vi "Set Center-Span.vi"() -> ()   [LabVIEW 2012, in "Microwave.lvclass"]
doc: "Sets the center and span (or start and stop) frequencies for a microwave sweep."
uses:
  Microwave.lvclass
  Microwave.lvclass/Microwave.ctl
  Math Operations/To Center and Span (frequency).vi
  Math Operations/To Start and Stop (frequency).vi
  Agilent PSG MXG Series/Agilent PSG MXG Series.lvlib
panel:
  in  "Adjust":bool
  in  "Distance from center\n(+/- # of boxes)":dbl
  in  "Width of scan\n(# of boxes)":dbl
  out "Ready when\nblinking":bool
  out "Dwell":dbl[unit]=0.052000000000000005 caption="Steps"
  in  "Dwell Set":dbl[unit]=0.001
  out "Steps":i32=52
  out "Power":dbl=23.0
  in  "Steps Set":i32=101
  in  "Power Set":dbl=23.0
  out "Current Amplitude Mode":enum16{"Fixed", "Stepped Sweep", "List Sweep"}(ring)
  out "Current Frequency Mode":T1(ring)
  out "error out":errorcluster
  in  "Copy actual to set":bool
  in  "Populate fields with member data":bool
  out "Fake Microwave out":refnum<class "Microwave.lvclass">
  in  "error in (no error)":errorcluster
  in  "Fake Microwave in":refnum<class "Microwave.lvclass">
  out "Stop":dbl[unit] caption="Center"
  in  "Stop Set":dbl[unit]
  out "Start":dbl[unit] caption="Center"
  in  "Start Set":dbl[unit]
  in  "Read to Control":bool
  in  "Read":bool
  out "Span":dbl[unit]
  out "Center":dbl[unit]
  in  "Span Set":dbl[unit] caption="Span"
  in  "Center Set":dbl[unit] caption="Center"
  in  "Rf On/Off":bool caption="RF On/Off"
  in  "Exit":bool
  in  "Set":bool
  # "Set Center and Span\nfor Freq Sweep"
  # "For info purposes:"
  # "dBm"
  # "ms"
  # "GHz"
  # "GHz"
  # "GHz"
  # "GHz"
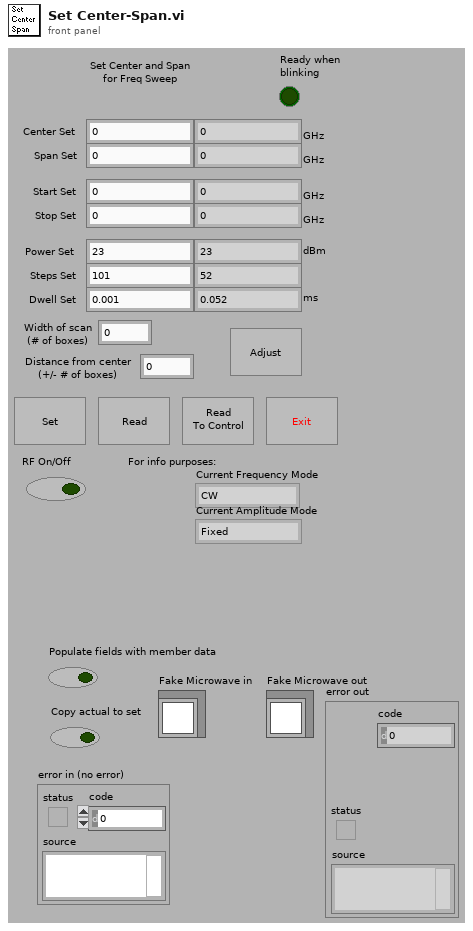
[diagram p1: front panel]
types:
  T1 = enum16{"CW", "Fixed", "Stepped Sweep", "List Sweep"}
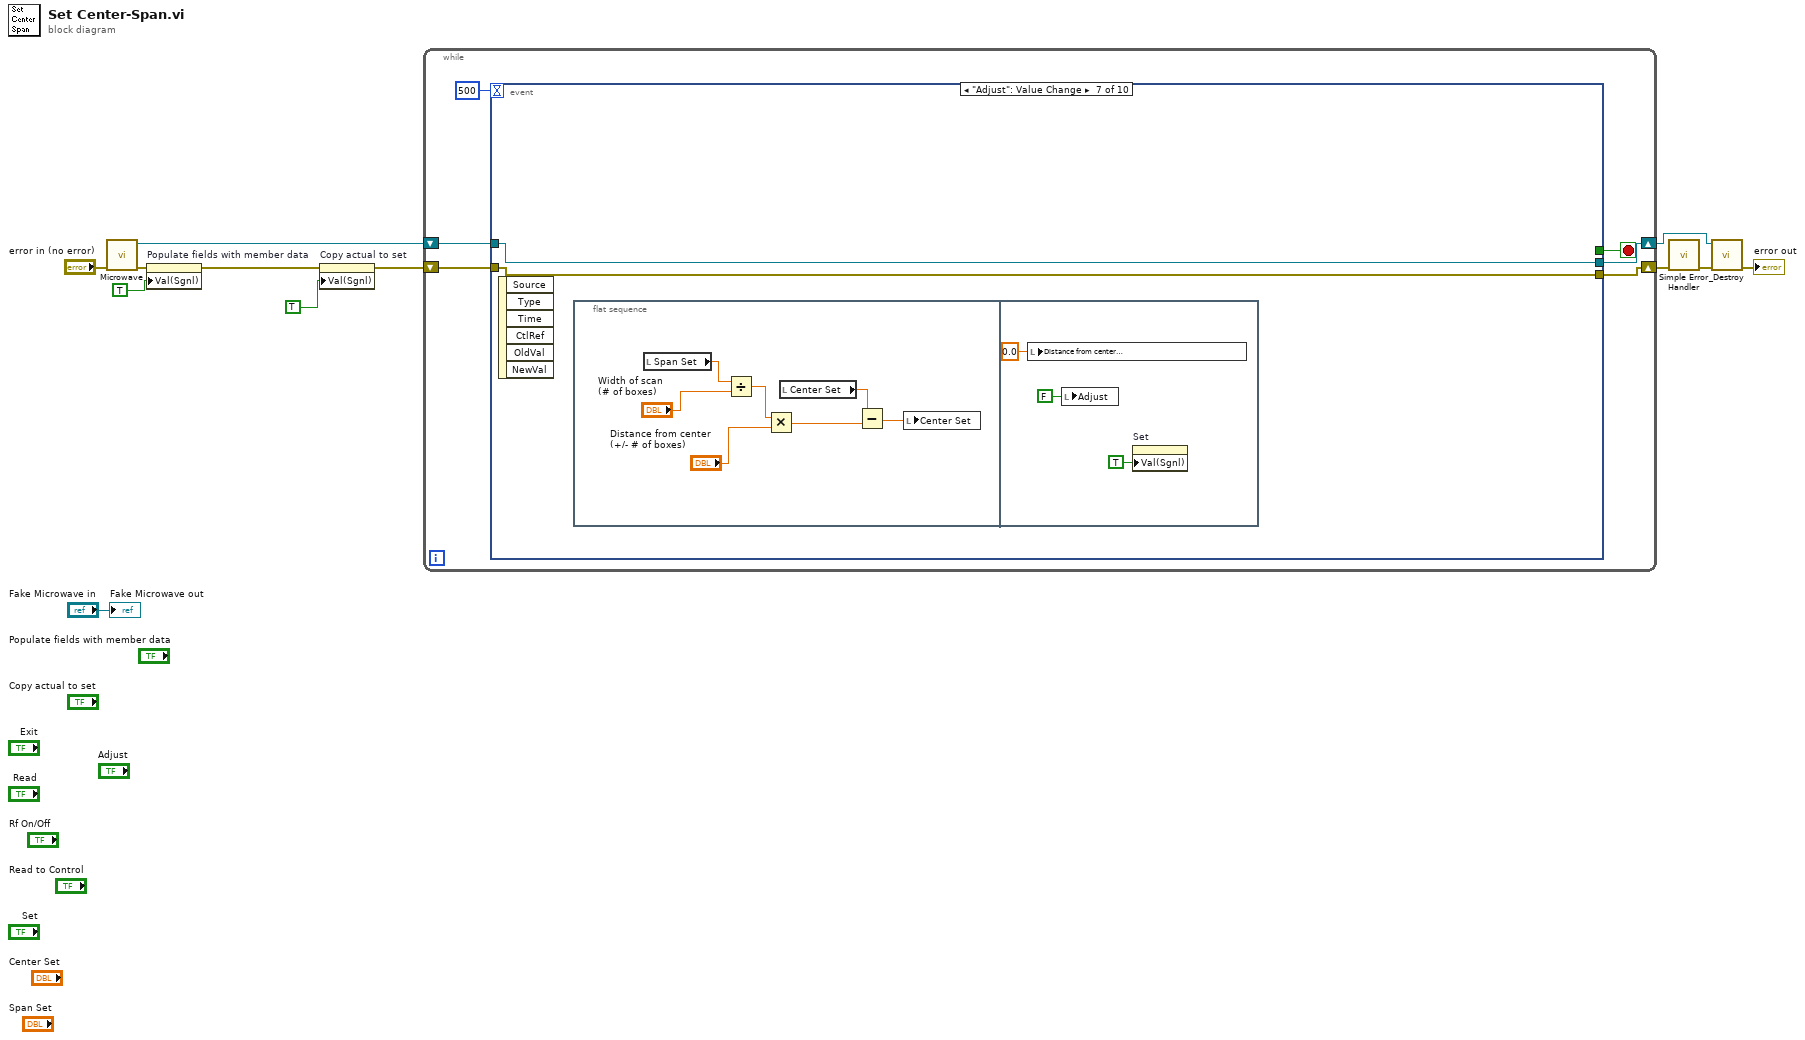
[diagram p0: block diagram]
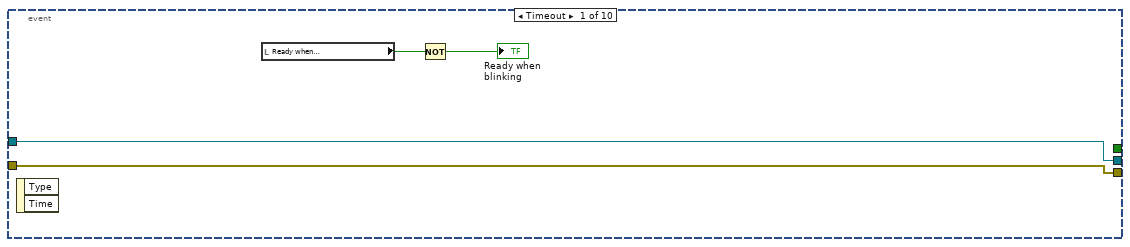
[diagram p2: hidden frame]
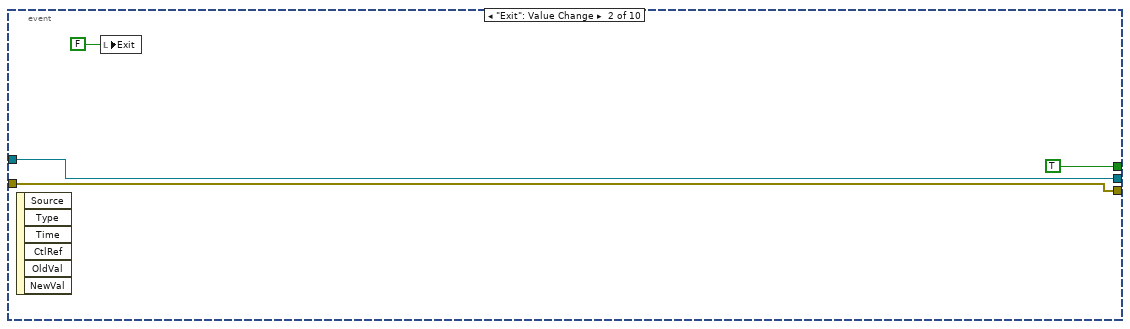
[diagram p3: hidden frame]
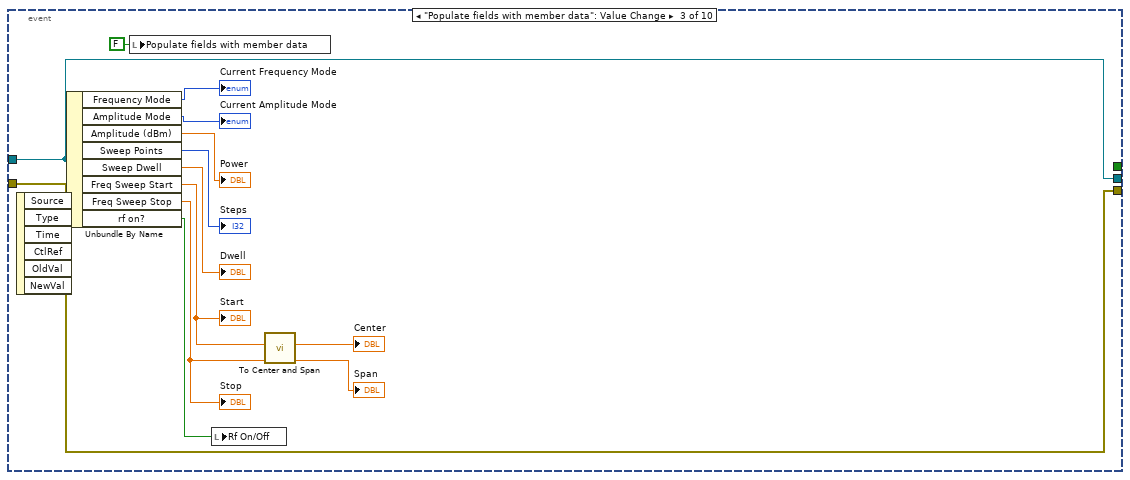
[diagram p4: hidden frame]
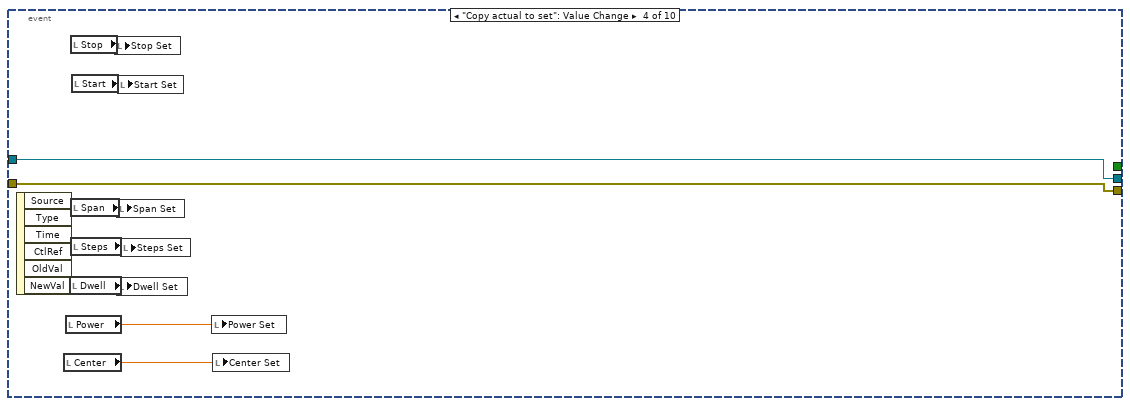
[diagram p5: hidden frame]
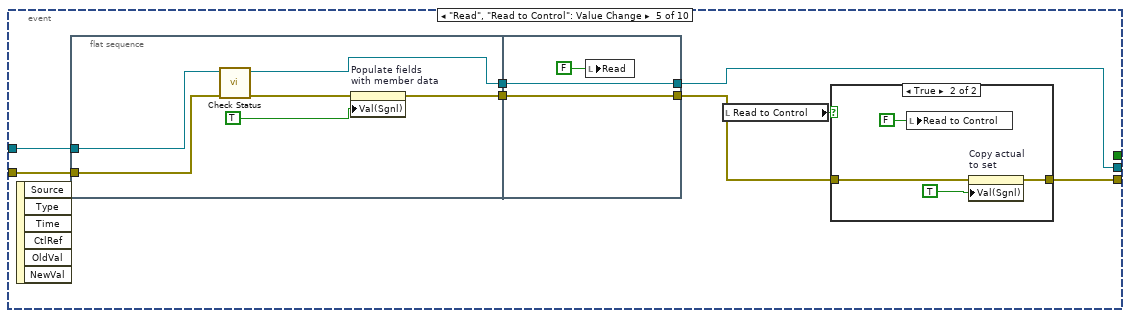
[diagram p6: hidden frame]
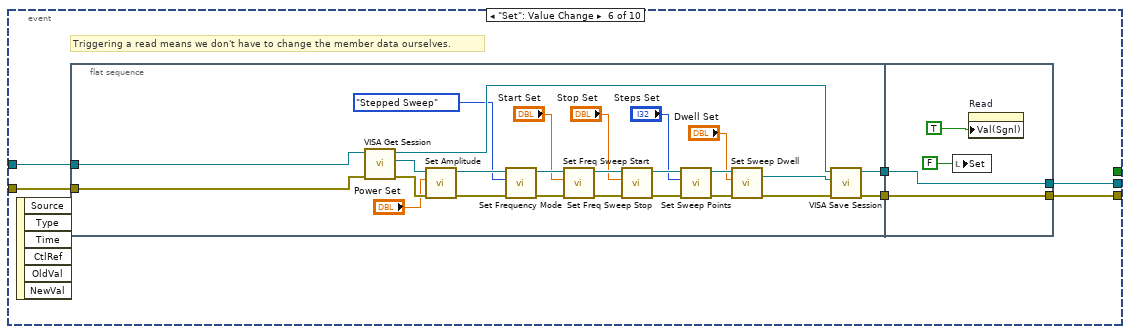
[diagram p8: hidden frame]
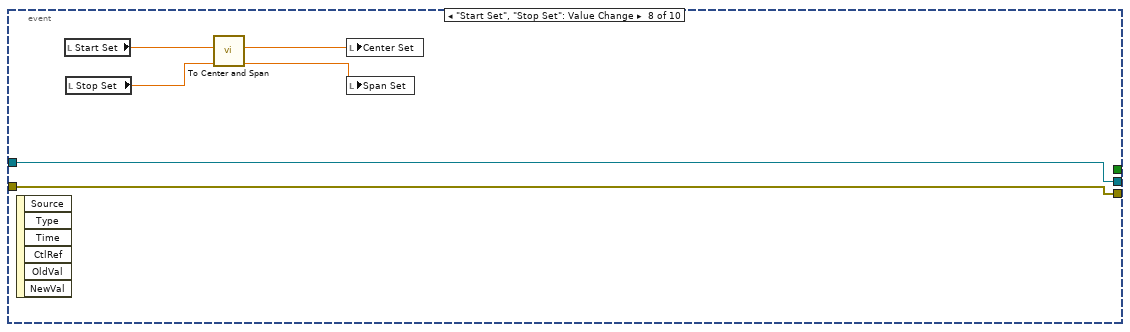
[diagram p9: hidden frame]
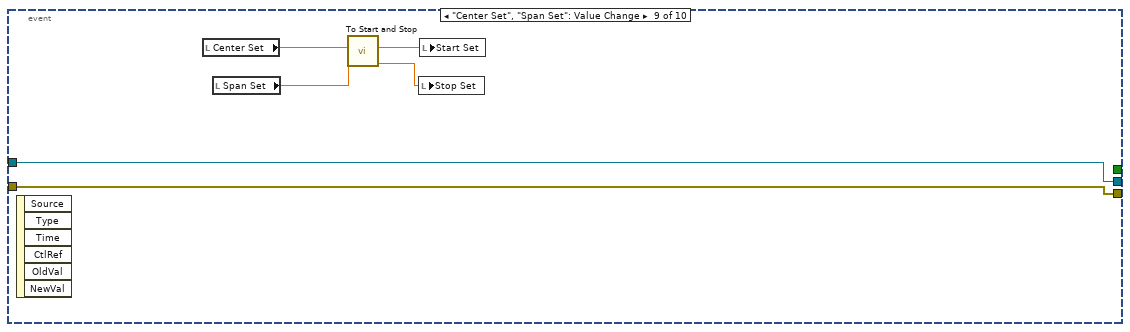
[diagram p10: hidden frame]
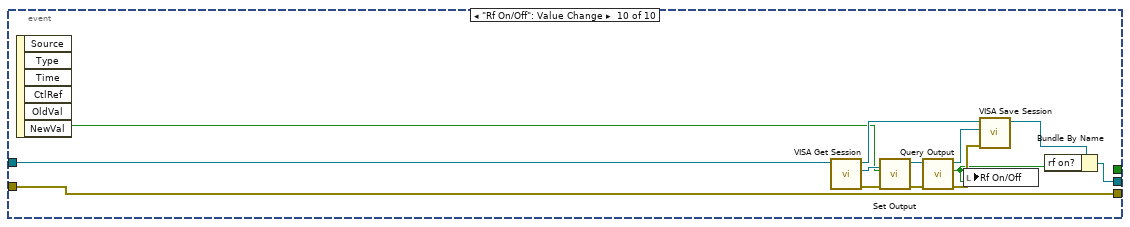
[diagram p11: hidden frame]
diagram:
  n1 = call "Microwave.vi"("error in (no error)"="error in (no error)") -> ("error out"=w9:errorcluster, "Microwave out"=w2:refnum<class "Microwave.lvclass">)  [unwired: 9 out]
  n2 = property on="Populate fields with member data" class="Bool (strict)"(error in=w9, "Val(Sgnl)"=TRUE ("Value (Signaling)")) -> (error out=w8:errorcluster)  [unwired: 1 in, 1 out]
  n3 = property on="Copy actual to set" class="Bool (strict)"(error in=w8, "Val(Sgnl)"=TRUE ("Value (Signaling)")) -> (error out=w1:errorcluster)  [unwired: 1 in, 1 out]
  n4 = while {
    shift-right: [w16] -> w3
    shift-left: w2 -> [w15]
    shift-right: [w17] -> w4
    shift-left: w1 -> [w14]
    stop <- w18 stop-if-true
    n5 = event shown="[6] \"Adjust\": Value Change" {
      selector: _ -> [_ _ _ _ _ _ _ _ _ _]
      dyn-events: _ -> [_ _ _ _ _ _ _ _ _ _]
      timeout: 500 -> [_ _ _ _ _ _ _ _ _ _]
      tunnel: [_ TRUE _ _ _ _ _ _ _ _] -> w18
      tunnel: [w21 w23 w39 w47 w50 w74 w107 w120 w124 w142] -> w17
      tunnel: w14 -> [w21 w23 w39 w47 w53 w75 w107 w120 w124 w142]
      tunnel: [w22 w24 w38 w48 w54 w72 w106 w121 w125 w132] -> w16
      tunnel: w15 -> [w22 w24 w38 w48 w55 w76 w106 w121 w125 w133]
      event Timeout {
        n6 = event-data() -> ()  [unwired: 3 out]
        n7 = local read "Ready when\nblinking"() -> (w19:bool)
        n8 = Not(x=w19) -> (.not. x?=→"Ready when\nblinking":bool)
      }
      event "Exit": Value Change {
        n9 = event-data() -> ()  [unwired: 7 out]
        n10 = local write "Exit"(FALSE ("Exit")) -> ()
      }
      event "Populate fields with member data": Value Change {
        n11 = event-data() -> ()  [unwired: 7 out]
        n12 = Unbundle By Name(w38) -> ("Frequency Mode"=→"Current Frequency Mode":u16, "Amplitude Mode"=→"Current Amplitude Mode":u16, "Amplitude (dBm)"=→"Power":dbl, "Sweep Points"=→"Steps":i32, "Sweep Dwell"=→"Dwell":dbl[unit], "Freq Sweep Start"=w32:dbl[unit], "Freq Sweep Stop"=w31:dbl[unit], "rf on?"=w28:bool)
        "Start" <- w32
        "Stop" <- w31
        n13 = local write "Populate fields with member data"(FALSE ("Populate fields with member data")) -> ()
        n14 = local write "Rf On/Off"(w28) -> ()
        n15 = call-poly "To Center and Span.vi"("stop"=w31, "start"=w32) -> ("span"=→"Span":dbl[unit], "center"=→"Center":dbl[unit])  [unwired: 4 out]
      }
      event "Copy actual to set": Value Change {
        n16 = event-data() -> ()  [unwired: 7 out]
        n17 = local read "Center"() -> (w46:dbl[unit])
        n18 = local read "Power"() -> (w42:dbl)
        n19 = local read "Dwell"() -> (w40:dbl[unit])
        n20 = local read "Stop"() -> (w43:dbl[unit])
        n21 = local read "Span"() -> (w45:dbl[unit])
        n22 = local read "Steps"() -> (w41:i32)
        n23 = local read "Start"() -> (w44:dbl[unit])
        n24 = local write "Stop Set"(w43) -> ()
        n25 = local write "Span Set"(w45) -> ()
        n26 = local write "Dwell Set"(w40) -> ()
        n27 = local write "Start Set"(w44) -> ()
        n28 = local write "Steps Set"(w41) -> ()
        n29 = local write "Power Set"(w42) -> ()
        n30 = local write "Center Set"(w46) -> ()
      }
      event "Read", "Read to Control": Value Change {
        n31 = event-data() -> ()  [unwired: 7 out]
        n32 = flat-sequence {
          tunnel: w55 -> [w62]
          tunnel: w53 -> [w60]
          tunnel: [w61] -> w52
          tunnel: [w57] -> w51
          tunnel: [w64] -> w49
          tunnel: [w65] -> w54
          tunnel: w52 -> [w65]
          tunnel: w51 -> [w64]
          frame #0 {
            n33 = call-dynamic "Check Status.vi"("error in (no error)"=w60, "Microwave in"=w62) -> ("error out"=w58:errorcluster, "Microwave out"=w61:refnum<class "Microwave.lvclass">)  [unwired: 8 out]
            n34 = property on="Populate fields \nwith member data" class="Bool (strict)"(error in=w58, "Val(Sgnl)"=TRUE ("Value (Signaling)")) -> (error out=w57:errorcluster)  [unwired: 1 in, 1 out]
          }
          frame #1 {
            n35 = local write "Read"(FALSE ("Read")) -> ()
          }
        }
        n36 = local read "Read to Control"() -> (w56:bool)
        n37 = case shown="True" w56 {
          tunnel: w49 -> [w66 w69]
          tunnel: [w66 w68] -> w50
          frame False {
          }
          frame True {
            n38 = local write "Read to Control"(FALSE ("Read to Control")) -> ()
            n39 = property on="Copy actual \nto set" class="Bool (strict)"(error in=w69, "Val(Sgnl)"=TRUE ("Value (Signaling)")) -> (error out=w68:errorcluster)  [unwired: 1 in, 1 out]
          }
        }
      }
      event "Set": Value Change {
        # "Triggering a read means we don't have to change the member data ourselves."
        n40 = event-data() -> ()  [unwired: 7 out]
        n41 = flat-sequence {
          tunnel: w76 -> [w101]
          tunnel: w75 -> [w85]
          tunnel: [w84] -> w73
          tunnel: [w83] -> w71
          tunnel: w73 -> [w104]
          tunnel: w71 -> [w103]
          tunnel: [w104] -> w74
          tunnel: [w103] -> w72
          frame #0 {
            n42 = call-dynamic "VISA Get Session.vi"("error in (no error)"=w85, "Instrument.lvclass in"=w101) -> ("error out"=w92:errorcluster, "VISA Resource Name"=w99:refnum<visa-resource-name>, "Instrument.lvclass out"=w100:refnum<class "Microwave.lvclass">)  [unwired: 7 out]
            n43 = call "Set Amplitude.vi"("error in (no error)"=w92, "Amplitude (dBm)"="Power Set", "VISA resource name"=w99) -> ("error out"=w91:errorcluster, "VISA resource name out"=w98:refnum<visa-resource-name>)  [unwired: 7 out]
            n44 = call "Set Frequency Mode.vi"("error in (no error)"=w91, "Frequency Mode"=T1."Stepped Sweep", "VISA resource name"=w98) -> ("error out"=w90:errorcluster, "VISA resource name out"=w97:refnum<visa-resource-name>)  [unwired: 7 out]
            n45 = call "Set Freq Sweep Start.vi"("error in (no error)"=w90, "Frequency Sweep Start"="Start Set", "VISA resource name"=w97) -> ("error out"=w89:errorcluster, "VISA resource name out"=w96:refnum<visa-resource-name>)  [unwired: 7 out]
            n46 = call "Set Freq Sweep Stop.vi"("error in (no error)"=w89, "Frequency Sweep Stop"="Stop Set", "VISA resource name"=w96) -> ("error out"=w88:errorcluster, "VISA resource name out"=w95:refnum<visa-resource-name>)  [unwired: 7 out]
            n47 = call "Set Sweep Points.vi"("error in (no error)"=w88, "Number of Sweep Points"="Steps Set", "VISA resource name"=w95) -> ("error out"=w87:errorcluster, "VISA resource name out"=w94:refnum<visa-resource-name>)  [unwired: 7 out]
            n48 = call "Set Sweep Dwell.vi"("error in (no error)"=w87, "Sweep Dwell Time"="Dwell Set", "VISA resource name"=w94) -> ("error out"=w86:errorcluster, "VISA resource name out"=w93:refnum<visa-resource-name>)  [unwired: 7 out]
            n49 = call-dynamic "VISA Save Session.vi"("error in (no error)"=w86, "VISA Resource Name"=w93, "Instrument.lvclass in"=w100) -> ("error out"=w84:errorcluster, "Instrument.lvclass out"=w83:refnum<class "Microwave.lvclass">)  [unwired: 7 out]
          }
          frame #1 {
            n50 = local write "Set"(FALSE ("Set")) -> ()
            n51 = property on="Read" class="Bool (strict)"("Val(Sgnl)"=TRUE ("Value (Signaling)")) -> ()  [unwired: 2 in, 2 out]
          }
        }
      }
      event "Adjust": Value Change {
        n52 = event-data() -> ()  [unwired: 7 out]
        n53 = flat-sequence {
          frame #0 {
            n54 = local read "Span Set"() -> (w108:dbl[unit])
            n55 = Divide(x=w108, y="Width of scan\n(# of boxes)") -> (x/y=w110:dbl[unit])
            n56 = Multiply(x=w110, y="Distance from center\n(+/- # of boxes)") -> (x*y=w113:dbl[unit])
            n57 = local read "Center Set"() -> (w112:dbl[unit])
            n58 = Subtract(x=w112, y=w113) -> (x-y=w114:dbl[unit])
            n59 = local write "Center Set"(w114) -> ()
          }
          frame #1 {
            n60 = local write "Distance from center\n(+/- # of boxes)"(0.0 ("Distance from center\n(+/- # of boxes)")) -> ()
            n61 = local write "Adjust"(FALSE ("Adjust")) -> ()
            n62 = property on="Set" class="Bool (strict)"("Val(Sgnl)"=TRUE ("Value (Signaling)")) -> ()  [unwired: 2 in, 2 out]
          }
        }
      }
      event "Start Set", "Stop Set": Value Change {
        n63 = event-data() -> ()  [unwired: 7 out]
        n64 = local read "Start Set"() -> (w119:dbl[unit])
        n65 = local read "Stop Set"() -> (w118:dbl[unit])
        n66 = call-poly "To Center and Span.vi"("stop"=w118, "start"=w119) -> ("span"=w122:dbl[unit], "center"=w123:dbl[unit])  [unwired: 4 out]
        n67 = local write "Center Set"(w123) -> ()
        n68 = local write "Span Set"(w122) -> ()
      }
      event "Center Set", "Span Set": Value Change {
        n69 = event-data() -> ()  [unwired: 7 out]
        n70 = local read "Center Set"() -> (w129:dbl[unit])
        n71 = local read "Span Set"() -> (w128:dbl[unit])
        n72 = call-poly "To Start and Stop.vi"("span"=w128, "center"=w129) -> ("stop"=w126:dbl[unit], "start"=w127:dbl[unit])  [unwired: 4 out]
        n73 = local write "Stop Set"(w126) -> ()
        n74 = local write "Start Set"(w127) -> ()
      }
      event "Rf On/Off": Value Change {
        n75 = event-data() -> ("NewVal"=w130:bool)  [unwired: 6 out]
        n76 = call-dynamic "VISA Get Session.vi"("Instrument.lvclass in"=w133) -> ("error out"=w140:errorcluster, "VISA Resource Name"=w141:refnum<visa-resource-name>, "Instrument.lvclass out"=w139:refnum<class "Microwave.lvclass">)  [unwired: 1 in, 7 out]
        n77 = call "Set Output.vi"("error in (no error)"=w140, "Output On"=w130, "VISA resource name"=w141) -> ("error out"=w136:errorcluster, "VISA resource name out"=w138:refnum<visa-resource-name>)  [unwired: 7 out]
        n78 = call "Query Output.vi"("error in (no error)"=w136, "VISA resource name"=w138) -> ("error out"=w135:errorcluster, "Output On?"=w131:bool, "VISA resource name out"=w137:refnum<visa-resource-name>)  [unwired: 7 out]
        n79 = local write "Rf On/Off"(w131) -> ()
        n80 = call-dynamic "VISA Save Session.vi"("error in (no error)"=w135, "VISA Resource Name"=w137, "Instrument.lvclass in"=w139) -> ("Instrument.lvclass out"=w134:refnum<class "Microwave.lvclass">)  [unwired: 8 out]
        n81 = Bundle By Name(cluster=w134, "rf on?"=w131) -> (w132:refnum<class "Microwave.lvclass">)
      }
    }
  }
  n82 = call <vilib>:"Simple Error Handler.vi"("error in (no error)"=w4) -> ("error out"=w6:errorcluster)  [unwired: 1 in, 7 out]
  n83 = call-dynamic "_Destroy.vi"("error in (no error)"=w6, "Instrument in"=w3) -> ("error out"=→"error out":errorcluster)  [unwired: 9 out]
  "Fake Microwave out" <- "Fake Microwave in"
